vi "main.vi"() -> ()   [LabVIEW 2023, in "parent.lvclass"]
uses:
  parent/parent.lvclass
  <vilib>/ActorFramework/Message Queue/Message Queue.lvclass
  <vilib>/ActorFramework/Actor/Actor.lvclass
  <vilib>/ActorFramework/Stop Msg/Stop Msg.lvclass
  subpanel 2/subpanel 2.lvclass
  subpanel 3/subpanel 3.lvclass
  subpanel 1/subpanel 1.lvclass
  subpanel/subpanel (abstract).lvclass
  N:/VT LTT Project/Source Code/GUI/Reused Code/Subpanels Actor/subpanels/subpanel/subpanel (abstract).lvclass
  C:/Program Files/National Instruments/LabVIEW 2023/vi.lib/ActorFramework/Actor/Actor.lvclass
  N:/VT LTT Project/Source Code/GUI/Reused Code/Subpanels Actor/subpanels/subpanel 1/subpanel 1.lvclass
  N:/VT LTT Project/Source Code/GUI/Reused Code/Subpanels Actor/subpanels/subpanel 2/subpanel 2.lvclass
  N:/VT LTT Project/Source Code/GUI/Reused Code/Subpanels Actor/subpanels/subpanel 3/subpanel 3.lvclass
panel:
  in  "Add":bool
  in  "sub 3":bool
  in  "sub 2":bool
  in  "exit":bool
  in  "sub 1":bool
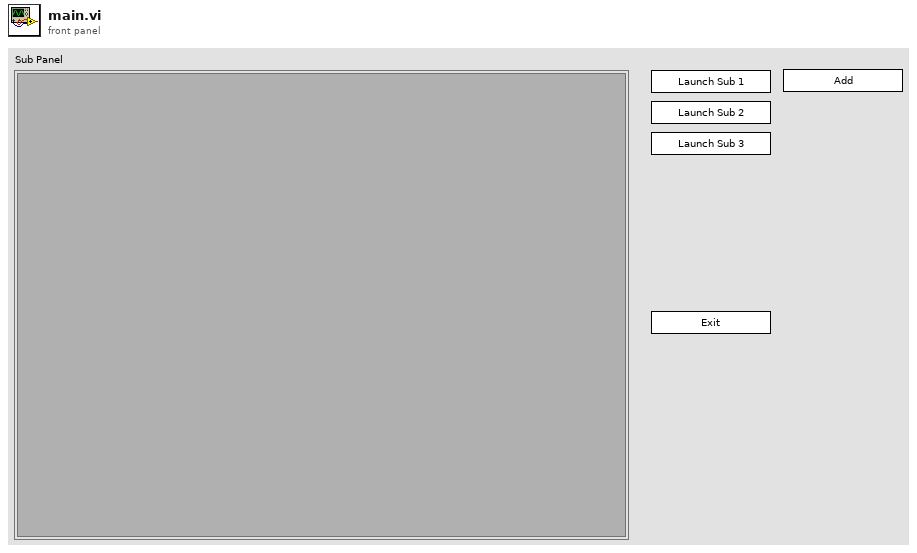
[diagram p1: front panel]
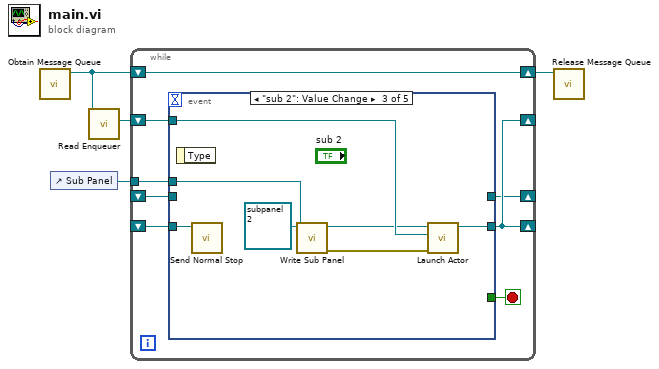
[diagram p0: block diagram]
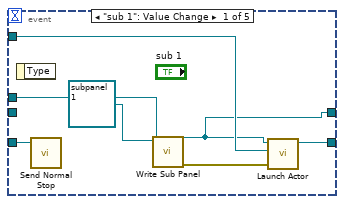
[diagram p2: hidden frame]
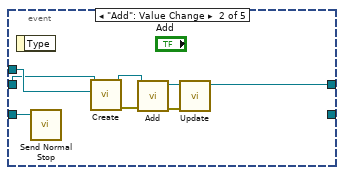
[diagram p3: hidden frame]
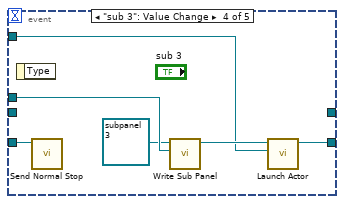
[diagram p4: hidden frame]
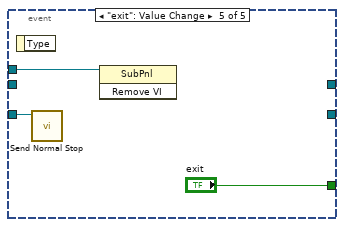
[diagram p5: hidden frame]
diagram:
  n1 = call <vilib>:"Obtain Message Queue.vi"() -> ("Message Queue"=w3:refnum<class "Message Queue.lvclass">)  [unwired: 10 in, 1 out]
  n2 = control-ref of="Sub Panel"() -> (w4:refnum<vi>)
  n3 = call <vilib>:"Read Enqueuer.vi"("Message Queue"=w3) -> ("Message Enqueuer"=w1:refnum<class "Message Enqueuer.lvclass">)  [unwired: 10 in]
  n4 = while {
    tunnel: w4 -> [w12]
    shift-right: [w7] -> _
    shift-left: _ -> [w10]
    shift-right: [w8] -> w2
    shift-left: w3 -> [w8]
    shift-right: [w7] -> _
    shift-left: w1 -> [w9]
    shift-right: [w6] -> _
    shift-left: _ -> [w5]
    stop <- w11 stop-if-true
    n5 = event shown="[2] \"sub 2\": Value Change" {
      selector: _ -> [_ _ _ _ _]
      dyn-events: _ -> [_ _ _ _ _]
      timeout: _ -> [_ _ _ _ _]
      tunnel: w12 -> [w19 w23 w34 w40 w42]
      tunnel: [_ _ _ _ "exit"] -> w11
      tunnel: [w18 _ w32 w37 _] -> w7
      tunnel: w10 -> [w13 w27 w31 w36 w41]
      tunnel: w9 -> [w17 _ w30 w35 _]
      tunnel: [w16 w24 _ _ _] -> w6
      tunnel: w5 -> [_ w22 _ _ _]
      event "sub 1": Value Change {
        n6 = event-data() -> ()  [unwired: 1 in, 1 out]
        n7 = call <vilib>:"Send Normal Stop.vi"("Message Enqueuer"=w13) -> ()  [unwired: 10 in, 1 out]
        n8 = call-dynamic "Write Sub Panel.vi"("Sub Panel"=w19, "subpanel_abstract in"=refnum<class "subpanel 1.lvclass"> refnum ("subpanel 1.lvclass")) -> ("error out"=w15:errorcluster, "subpanel_abstract out"=w16:refnum<class "subpanel 1.lvclass">)  [unwired: 8 in]
        n9 = call <vilib>:"Launch Actor.vi"("error in (no error)"=w15, "Actor-to-Caller Enqueuer"=w17, "Actor"=w16) -> ("Caller-To-Actor Enqueuer"=w18:refnum<class "Message Enqueuer.lvclass">)  [unwired: 7 in, 1 out]
      }
      event "Add": Value Change {
        n10 = event-data() -> ()  [unwired: 1 in, 1 out]
        n11 = call <vilib>:"Send Normal Stop.vi"("Message Enqueuer"=w27) -> ()  [unwired: 10 in, 1 out]
        n12 = call "Create.vi"("reference"=w23, "subpanel (abstract) in"=w22) -> ("error out"=w20:errorcluster, "subpanel (abstract) out"=w21:refnum<class "subpanel (abstract).lvclass">)  [unwired: 7 in, 1 out]
        n13 = call-dynamic "Add.vi"("error in (no error)"=w20, "subpanel (abstract) in"=w21) -> ("error out"=w26:errorcluster, "subpanel (abstract) out"=w25:refnum<class "subpanel (abstract).lvclass">)  [unwired: 8 in]
        n14 = call-dynamic "Update.vi"("error in (no error)"=w26, "subpanel (abstract) in"=w25) -> ("subpanel (abstract) out"=w24:refnum<class "subpanel (abstract).lvclass">)  [unwired: 8 in, 1 out]
      }
      event "sub 2": Value Change {
        n15 = event-data() -> ()  [unwired: 1 in, 1 out]
        n16 = call <vilib>:"Send Normal Stop.vi"("Message Enqueuer"=w31) -> ()  [unwired: 10 in, 1 out]
        n17 = call-dynamic "Write Sub Panel.vi"("Sub Panel"=w34, "subpanel_abstract in"=refnum<class "subpanel 2.lvclass"> refnum ("subpanel_abstract.lvclass")) -> ("error out"=w28:errorcluster, "subpanel_abstract out"=w29:refnum<class "subpanel 2.lvclass">)  [unwired: 8 in]
        n18 = call <vilib>:"Launch Actor.vi"("error in (no error)"=w28, "Actor-to-Caller Enqueuer"=w30, "Actor"=w29) -> ("Caller-To-Actor Enqueuer"=w32:refnum<class "Message Enqueuer.lvclass">)  [unwired: 7 in, 1 out]
      }
      event "sub 3": Value Change {
        n19 = event-data() -> ()  [unwired: 1 in, 1 out]
        n20 = call <vilib>:"Send Normal Stop.vi"("Message Enqueuer"=w36) -> ()  [unwired: 10 in, 1 out]
        n21 = call-dynamic "Write Sub Panel.vi"("Sub Panel"=w40, "subpanel_abstract in"=refnum<class "subpanel 3.lvclass"> refnum ("subpanel_abstract.lvclass")) -> ("subpanel_abstract out"=w38:refnum<class "subpanel 3.lvclass">)  [unwired: 8 in, 1 out]
        n22 = call <vilib>:"Launch Actor.vi"("Actor-to-Caller Enqueuer"=w35, "Actor"=w38) -> ("Caller-To-Actor Enqueuer"=w37:refnum<class "Message Enqueuer.lvclass">)  [unwired: 8 in, 1 out]
      }
      event "exit": Value Change {
        n23 = event-data() -> ()  [unwired: 1 in, 1 out]
        n24 = call <vilib>:"Send Normal Stop.vi"("Message Enqueuer"=w41) -> ()  [unwired: 10 in, 1 out]
        n25 = invoke class="SubPnl" method="Remove VI"(reference=w42) -> ()  [unwired: 2 in, 3 out]
      }
    }
  }
  n26 = call <vilib>:"Release Message Queue.vi"("Message Queue"=w2) -> ()  [unwired: 9 in, 2 out]
